vi "Serial Write Read.vi"(8 "error in (no error)":errorcluster, 10 "Write Buffer":string, 11 "VISA resource name":refnum<visa-resource-name>) -> (0 "error out":errorcluster, 2 "Read Buffer":string, 3 "VISA resource name out":refnum<visa-resource-name>)   [LabVIEW 2018, in "XP Power PLS600.lvlib"]
doc: "Sends the data input in <B>Write Buffer</B> to the instrument and waits for the response, which includes the termination character. For query/status commands, the response will be returned in <B>Read Buffer</B>. For action commands that do not return a response, <B>Read Buffer</B> will be blank, however, since the instrument still responds with a LF termination character, when this VI returns the instrument has successfully received the command."
uses:
  XP Power PLS600.lvlib
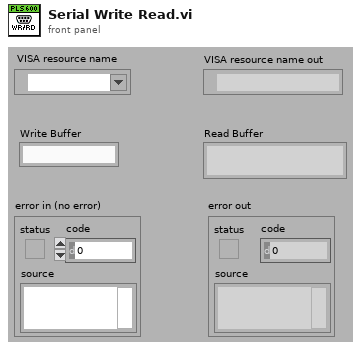
[diagram p1: front panel]
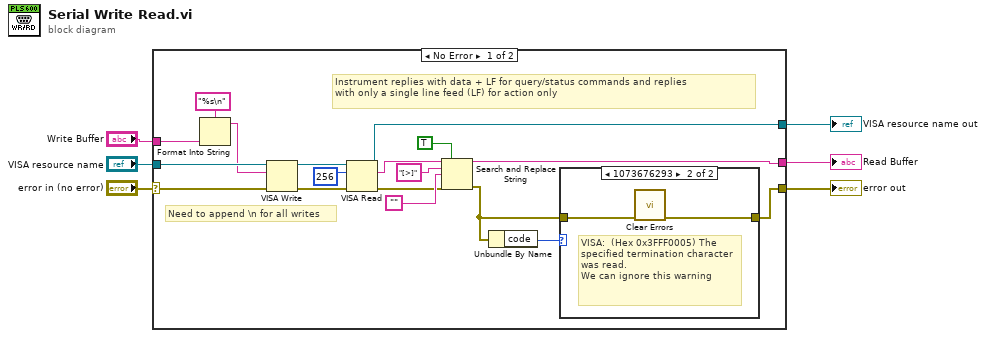
[diagram p0: block diagram]
diagram:
  n1 = case shown="No Error" "error in (no error)" {
    selector: "error in (no error)" -> [w16 w29]
    tunnel: "VISA resource name" -> [w21 w28]
    tunnel: [w14 w29] -> w5
    tunnel: [w20 w28] -> w1
    tunnel: [w8 _] -> w4
    tunnel: "Write Buffer" -> [w18 _]
    frame No Error {
      # "Need to append \\n for all writes"
      # "Instrument replies with data + LF for query/status commands and replies \nwith only a single line feed (LF) for action only"
      n2 = Format Into String(format string="%s\n", w18) -> (resulting string=w17:string)  [unwired: 2 in, 1 out]
      n3 = VISA Write(VISA resource name=w21, write buffer=w17, error in (no error)=w16) -> (VISA resource name out=w23:refnum<visa-resource-name>, error out=w22:errorcluster)  [unwired: 1 out]
      n4 = VISA Read(VISA resource name=w23, byte count=u32 256, error in (no error)=w22) -> (VISA resource name out=w20:refnum<visa-resource-name>, read buffer=w9:string, error out=w10:errorcluster)  [unwired: 1 out]
      n5 = Search and Replace String(replace all?=TRUE ("replace all? (F)"), input string=w9, search string="[>]" ("regular expression"), replace string="", error in=w10) -> (result string=w8:string, error out=w7:errorcluster)  [unwired: 3 in, 2 out]
      n6 = Unbundle By Name(w7) -> ("code"=w15:i32)
      n7 = case shown="1073676293" w15 {
        tunnel: w7 -> [w25 w27]
        tunnel: [w25 w26] -> w14
        frame 0, Default {
        }
        frame 1073676293 {
          # "VISA:  (Hex 0x3FFF0005) The specified termination character was read.\nWe can ignore this warning"
          n8 = call <vilib>:"Clear Errors.vi"("error in (no error)"=w27) -> ("error out"=w26:errorcluster)  [unwired: 5 in, 1 out]
        }
      }
    }
    frame Error {
    }
  }
  "VISA resource name out" <- w1
  "error out" <- w5
  "Read Buffer" <- w4
